vi "test Parse Stream Set.vi"() -> (0 "error out":errorcluster, 2 "pass?":bool)   [LabVIEW 2019, in "RESP3 Tests.lvlib"]
uses:
  RESP3 Tests.lvlib
  RESP3/RESP3 Parser/RESP3 Parser.lvclass
  RESP3/types/RESP3 Type.ctl
  e6dd2cc8-9acc-4614-821b-38df5cde0bed.vi
  641257fe-6faf-45e9-83e6-5a5ed817c619.vi
  a7ea5d2a-efc5-4c2c-be3c-51ef07264278.vi
  531223f0-c2f5-4287-9115-8b7e737394d1.vi
  cd095cd9-fc4b-4fb7-9722-b19daafcaabf.vi
  RESP3/types/RESP3 data type attribute.vi
  RESP3/RESP3.lvlib
panel:
  out "RESP3 Value":variant
  out "finished?":bool
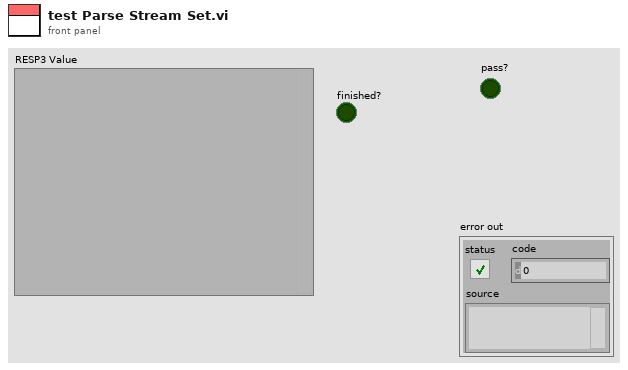
[diagram p1: front panel]
types:
  T1 = typedef "RESP3.lvlib/RESP3 Type.ctl" = enum8{"<0x00>", "<0x01>", "<0x02>", "<0x03>", "<0x04>", "<0x05>", "<0x06>", "<0x07>", "<0x08>", "<0x09>", "<0x0A>", "<0x0B>", "<0x0C>", "<0x0D>", "<0x0E>", "<0x0F>", "<0x10>", "<0x11>", "<0x12>", "<0x13>", "<0x14>", "<0x15>", "<0x16>", "<0x17>", "<0x18>", "<0x19>", "<0x1A>", "<0x1B>", "<0x1C>", "<0x1D>", "<0x1E>", "<0x1F>", "\" \"", "BLOB ERROR", "\"\"\"", "BOOLEAN", "BLOB", "MAP", "\"&\"", "\"'\"", "BIG NUMBER", "\")\"", "ARRAY", "STRING", "DOUBLE", "ERROR", "END", "\"/\"", "\"0\"", "\"1\"", "\"2\"", "\"3\"", "\"4\"", "\"5\"", "\"6\"", "\"7\"", "\"8\"", "\"9\"", "INTEGER", "STREAM", "\"<\"", "VERBATIM STRING", "PUSH", "\"?\"", "\"@\"", "\"A\"", "\"B\"", "\"C\"", "\"D\"", "\"E\"", "\"F\"", "\"G\"", "\"H\"", "\"I\"", "\"J\"", "\"K\"", "\"L\"", "\"M\"", "\"N\"", "\"O\"", "\"P\"", "\"Q\"", "\"R\"", "\"S\"", "\"T\"", "\"U\"", "\"V\"", "\"W\"", "\"X\"", "\"Y\"", "\"Z\"", "\"[\"", "\"\\\"", "\"]\"", "\"^\"", "NULL", "\"`\"", "\"a\"", "\"b\"", "\"c\"", "\"d\"", "\"e\"", "\"f\"", "\"g\"", "\"h\"", "\"i\"", "\"j\"", "\"k\"", "\"l\"", "\"m\"", "\"n\"", "\"o\"", "\"p\"", "\"q\"", "\"r\"", "\"s\"", "\"t\"", "\"u\"", "\"v\"", "\"w\"", "\"x\"", "\"y\"", "\"z\"", "\"{\"", "ATTRIBUTES", "\"}\"", "SET", "<0x7F>", "<0x80>", "<0x81>", "<0x82>", "<0x83>", "<0x84>", "<0x85>", "<0x86>", "<0x87>", "<0x88>", "<0x89>", "<0x8A>", "<0x8B>", "<0x8C>", "<0x8D>", "<0x8E>", "<0x8F>", "<0x90>", "<0x91>", "<0x92>", "<0x93>", "<0x94>", "<0x95>", "<0x96>", "<0x97>", "<0x98>", "<0x99>", "<0x9A>", "<0x9B>", "<0x9C>", "<0x9D>", "<0x9E>", "<0x9F>", "<0xA0>", "<0xA1>", "<0xA2>", "<0xA3>", "<0xA4>", "<0xA5>", "<0xA6>", "<0xA7>", "<0xA8>", "<0xA9>", "<0xAA>", "<0xAB>", "<0xAC>", "<0xAD>", "<0xAE>", "<0xAF>", "<0xB0>", "<0xB1>", "<0xB2>", "<0xB3>", "<0xB4>", "<0xB5>", "<0xB6>", "<0xB7>", "<0xB8>", "<0xB9>", "<0xBA>", "<0xBB>", "<0xBC>", "<0xBD>", "<0xBE>", "<0xBF>", "<0xC0>", "<0xC1>", "<0xC2>", "<0xC3>", "<0xC4>", "<0xC5>", "<0xC6>", "<0xC7>", "<0xC8>", "<0xC9>", "<0xCA>", "<0xCB>", "<0xCC>", "<0xCD>", "<0xCE>", "<0xCF>", "<0xD0>", "<0xD1>", "<0xD2>", "<0xD3>", "<0xD4>", "<0xD5>", "<0xD6>", "<0xD7>", "<0xD8>", "<0xD9>", "<0xDA>", "<0xDB>", "<0xDC>", "<0xDD>", "<0xDE>", "<0xDF>", "<0xE0>", "<0xE1>", "<0xE2>", "<0xE3>", "<0xE4>", "<0xE5>", "<0xE6>", "<0xE7>", "<0xE8>", "<0xE9>", "<0xEA>", "<0xEB>", "<0xEC>", "<0xED>", "<0xEE>", "<0xEF>", "<0xF0>", "<0xF1>", "<0xF2>", "<0xF3>", "<0xF4>", "<0xF5>", "<0xF6>", "<0xF7>", "<0xF8>", "<0xF9>", "<0xFA>", "<0xFB>", "<0xFC>", "<0xFD>", "<0xFE>"}
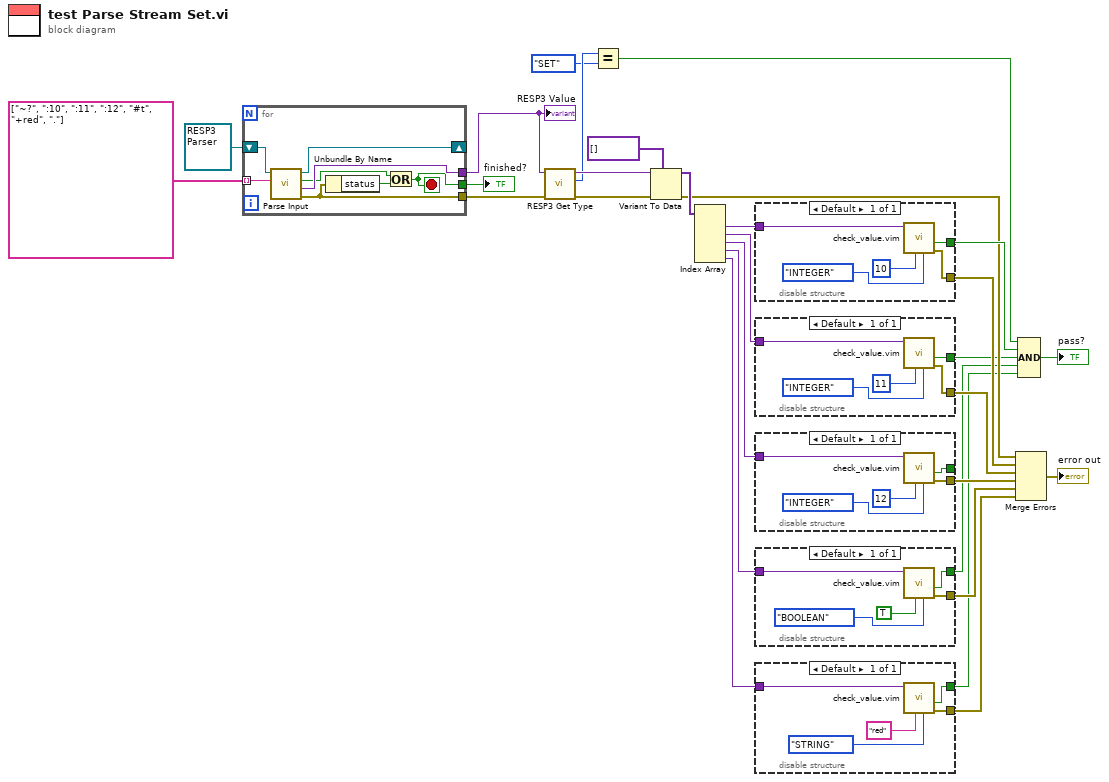
[diagram p0: block diagram]
diagram:
  n1 = for {
    shift-right: [w35] -> _
    shift-left: refnum<class "RESP3 Parser.lvclass"> refnum ("RESP3.lvlib:RESP3 Parser.lvclass") -> [w36]
    tunnel: string[] ["~?", ":10", ":11", ":12", "#t", "+red", "."] -> [w34] mode=indexing
    tunnel: [w33] -> w24
    tunnel: [w31] -> w26
    tunnel: [w29] -> w19
    stop <- w31 stop-if-true
    n2 = call-dynamic "Parse Input.vi"("input line"=w34, "RESP3 Parser in"=w36) -> ("error out"=w29:errorcluster, "RESP3 Value"=w33:variant, "finished?"=w32:bool, "RESP3 Parser out"=w35:refnum<class "RESP3 Parser.lvclass">)  [unwired: 6 in]
    n3 = Unbundle By Name(w29) -> ("status"=w30:bool)
    n4 = Or(x=w32, y=w30) -> (x .or. y?=w31:bool)
  }
  "finished?" <- w26
  "RESP3 Value" <- w24
  n5 = call "RESP3 Get Type.vi"("RESP3 Value in"=w24) -> ("RESP3 Type"=w22:T1, "RESP3 Value out"=w23:variant)  [unwired: 7 in, 2 out]
  n6 = Equal?(x=w22, y=RESP3_Type."SET") -> (x = y?=w20:bool)
  n7 = Variant To Data(error in=w19, type=variant[] [], Variant=w23) -> (data=w18:variant[], error out=w14:errorcluster)
  n8 = Index Array(array=w18) -> (element #1=w16:variant, element #2=w11:variant, element #3=w10:variant, element #4=w9:variant, element #5=w8:variant)  [unwired: 5 in]
  n9 = disable-structure shown="Default" {
    disable-tunnel: w16 -> [w41]
    disable-tunnel: [w38] -> w15
    disable-tunnel: [w37] -> w13
    frame Enabled {
      n10 = call "check_value.vim"("expected type"=RESP3_Type."INTEGER", "expected value"=10, "RESP3 Value"=w41) -> ("error out"=w37:errorcluster, "all OK?"=w38:bool)  [unwired: 5 in, 2 out]
    }
  }
  n11 = disable-structure shown="Default" {
    disable-tunnel: w11 -> [w46]
    disable-tunnel: [w43] -> w3
    disable-tunnel: [w42] -> w7
    frame Enabled {
      n12 = call "check_value.vim"("expected type"=RESP3_Type."INTEGER", "expected value"=11, "RESP3 Value"=w46) -> ("error out"=w42:errorcluster, "all OK?"=w43:bool)  [unwired: 5 in, 2 out]
    }
  }
  n13 = disable-structure shown="Default" {
    disable-tunnel: w10 -> [w51]
    disable-tunnel: [w48] -> _
    disable-tunnel: [w47] -> w6
    frame Enabled {
      n14 = call "check_value.vim"("expected type"=RESP3_Type."INTEGER", "expected value"=12, "RESP3 Value"=w51) -> ("error out"=w47:errorcluster, "all OK?"=w48:bool)  [unwired: 5 in, 2 out]
    }
  }
  n15 = disable-structure shown="Default" {
    disable-tunnel: w9 -> [w56]
    disable-tunnel: [w54] -> w2
    disable-tunnel: [w53] -> w5
    frame Enabled {
      n16 = call "check_value.vim"("expected type"=RESP3_Type."BOOLEAN", "expected value"=TRUE, "RESP3 Value"=w56) -> ("error out"=w53:errorcluster, "all OK?"=w54:bool)  [unwired: 5 in, 2 out]
    }
  }
  n17 = disable-structure shown="Default" {
    disable-tunnel: w8 -> [w61]
    disable-tunnel: [w59] -> w1
    disable-tunnel: [w58] -> w4
    frame Enabled {
      n18 = call "check_value.vim"("expected type"=RESP3_Type."STRING", "expected value"="red", "RESP3 Value"=w61) -> ("error out"=w58:errorcluster, "all OK?"=w59:bool)  [unwired: 5 in, 2 out]
    }
  }
  n19 = Merge Errors(w14, w13, w7, w6, w5, w4) -> (→"error out":errorcluster)
  n20 = Compound Arithmetic op=AND(w20, w15, w3, w2, w1) -> (→"pass?":bool)
